vi "Generate_SN.vi"(8 "error in (no error)":errorcluster caption="entrée d'erreur (pas d'erreur)", 11 "Class Creation_SN (Default) en entrée":refnum<class "Creation_SN Database (Default).lvclass">) -> (0 "error out":errorcluster caption="sortie d'erreur", 3 "Class Creation_SN (Default) en sortie":refnum<class "Creation_SN Database (Default).lvclass">)   [LabVIEW 2020, in "Library Instrument & Equipement.lvlib" / "Library Creation_SN.lvlib" / "Creation_SN Database (Default).lvclass"]
uses:
  Creation_SN Database (Default).lvclass
  Firebase/Source/Firebase Recovery_SN/Firebase Recovery_SN.lvclass
  C:/Users/ngarcin/OneDrive - Altyor/Standard TB/Class/Firebase/Source/Firebase Driver/Firebase Driver.lvclass
  Instrument/Instrument Firebase Altyor/Class Instrument Firebase Altyor.lvclass
  Creation_SN Database (Default).lvclass/Creation_SN Database (Default).ctl
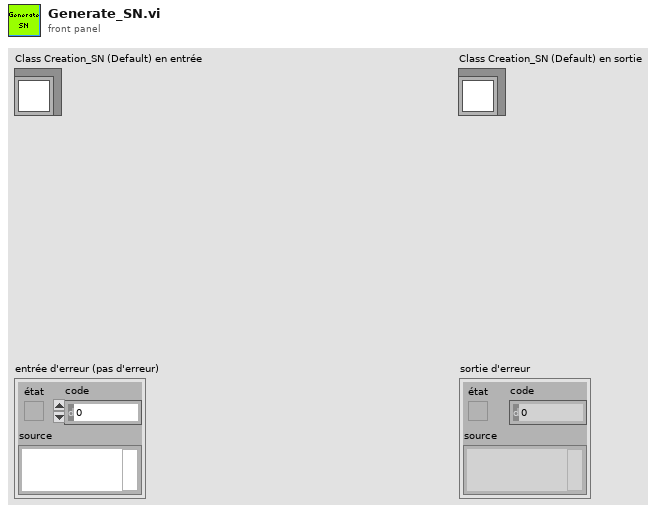
[diagram p1: front panel]
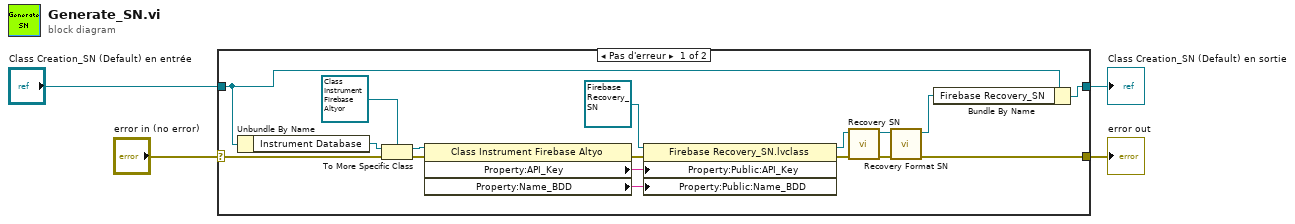
[diagram p0: block diagram]
diagram:
  n1 = case shown="Pas d'erreur" "error in (no error)" {
    selector: "error in (no error)" -> [w10 w23]
    tunnel: [w7 w23] -> w3
    tunnel: [w9 w22] -> w1
    tunnel: "Class Creation_SN (Default) en entrée" -> [w21 w22]
    frame No Error {
      n2 = Unbundle By Name(w21) -> ("Instrument Database"=w11:refnum<class "Class Instrument (Default).lvclass">)
      n3 = To More Specific Class(target class=refnum<class "Class Instrument Firebase Altyor.lvclass"> refnum ("Library Instruments.lvlib:Class Instrument Firebase Altyor.lvclass"), reference=w11, error in=w10) -> (specific class reference=w18:refnum<class "Class Instrument Firebase Altyor.lvclass">, error out=w19:errorcluster)
      n4 = property class="Class Instrument Firebase Altyo"(reference=w18, error in=w19) -> (error out=w16:errorcluster, "Property:API_Key"=w14:string, "Property:Name_BDD"=w13:string)  [unwired: 1 out]
      n5 = property class="Firebase Recovery_SN.lvclass"(reference=refnum<class "Firebase Recovery_SN.lvclass"> refnum ("Library FireBase.lvlib:Firebase Recovery_SN.lvclass"), error in=w16, "Property:Public:API_Key"=w14, "Property:Public:Name_BDD"=w13) -> (reference out=w12:refnum<class "Firebase Recovery_SN.lvclass">, error out=w15:errorcluster)
      n6 = call-dynamic "Recovery SN.vi"("error in (no error)"=w15, "Firebase Benches en entrée"=w12) -> ("error out"=w8:errorcluster, "Firebase Benches en sortie"=w6:refnum<class "Firebase Recovery_SN.lvclass">)  [unwired: 8 in]
      n7 = call-dynamic "Recovery Format SN.vi"("error in (no error)"=w8, "Firebase Benches en entrée"=w6) -> ("error out"=w7:errorcluster, "Firebase Benches en sortie"=w5:refnum<class "Firebase Recovery_SN.lvclass">)  [unwired: 8 in]
      n8 = Bundle By Name(cluster=w21, "Firebase Recovery_SN"=w5) -> (w9:refnum<class "Creation_SN Database (Default).lvclass">)
    }
    frame Error {
    }
  }
  "error out" <- w3
  "Class Creation_SN (Default) en sortie" <- w1
